vi "Stop Core.vi"(10 "final error code":i32, 11 "GUARDAR_CSV in":refnum<class "GUARDAR_CSV.lvclass">) -> (3 "GUARDAR_CSV out":refnum<class "GUARDAR_CSV.lvclass">)   [LabVIEW 2019, in "GUARDAR_CSV.lvlib" / "GUARDAR_CSV.lvclass"]
doc: "(<B>Filename</B>: Actor Framework.lvlib:Actor.lvclass:Stop Core.vi)\n\nDefines what the actor does before it stops. Use the <B>final error code</B> input to determine whether the actor shut down in response to an error.\n\nBy default, this method passes the Stop message along to all auto-stop nested actors. A descendant class may override this method to define additional behavior, such as shutting down any processes the actor initiated in its override of the Actor Core method."
uses:
  GUARDAR_CSV.lvclass
  <vilib>/ActorFramework/Actor/Actor.lvclass
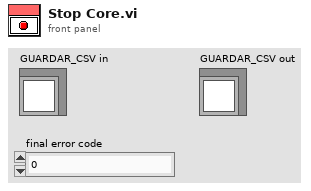
[diagram p1: front panel]
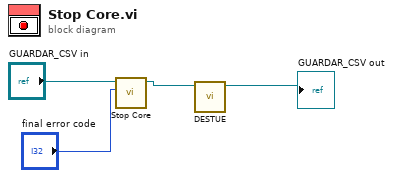
[diagram p0: block diagram]
diagram:
  n1 = call-parent "Stop Core.vi"("final error code"="final error code", "Actor in"="GUARDAR_CSV in") -> ("Actor out"=w2:refnum<class "GUARDAR_CSV.lvclass">)  [unwired: 9 in]
  n2 = call "DESTUE.vi"("GUARDAR_CSV in"=w2) -> ("GUARDAR_CSV out"=→"GUARDAR_CSV out":refnum<class "GUARDAR_CSV.lvclass">)  [unwired: 9 in, 1 out]
